vi "Test_uart.vi"() -> ()   [LabVIEW 2025]
uses:
  <vilib>/Instr/_visa.llb/VISA Configure Serial Port (Instr).vi
panel:
  in  "Caja engranes":sgl
  in  "Stop Button":bool
  out "Waveform Chart":cluster{"Número":sgl, "Número":sgl}(graph)
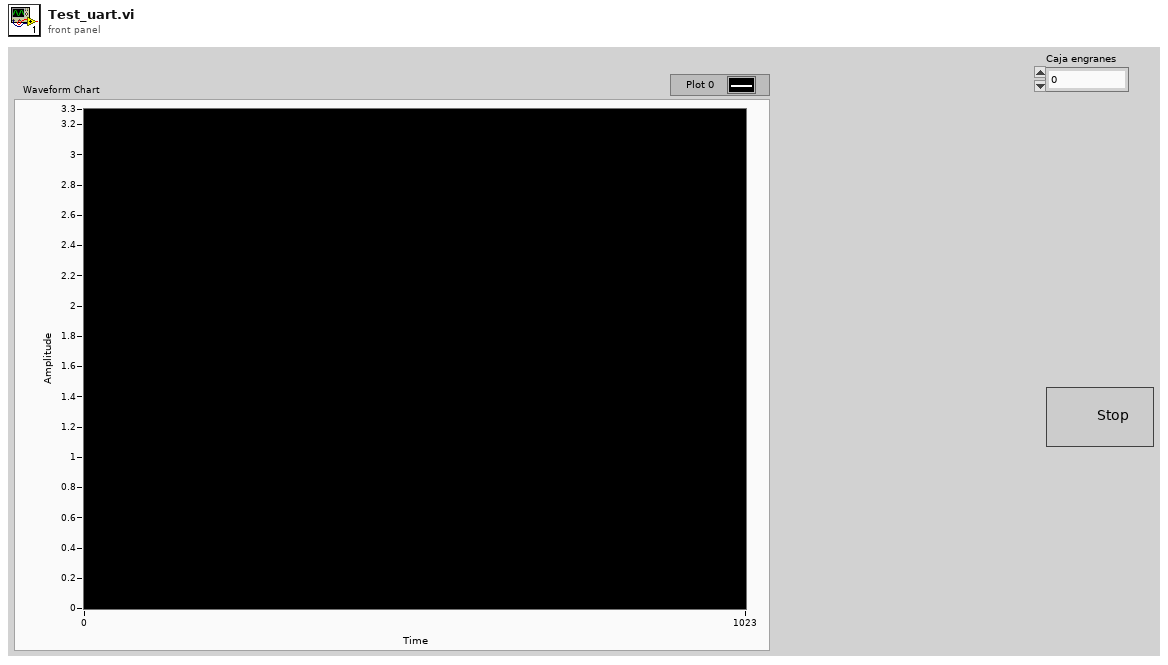
[diagram p1: front panel]
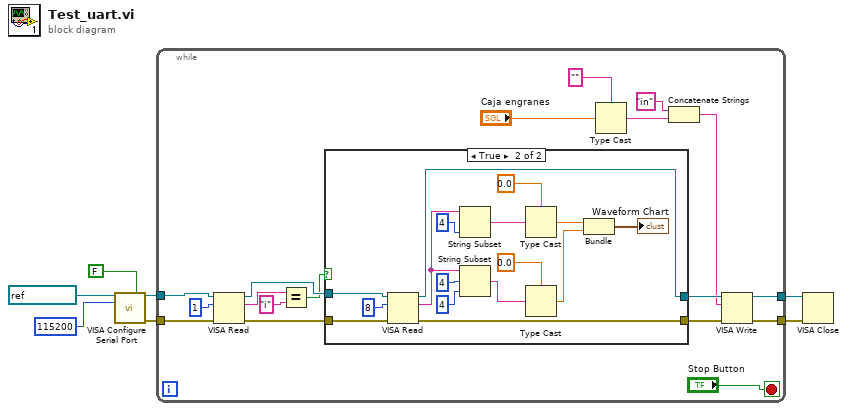
[diagram p0: block diagram]
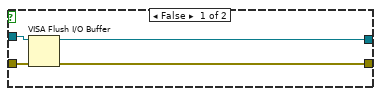
[diagram p2: hidden frame]
diagram:
  n1 = call-poly "VISA Configure Serial Port"("VISA resource name"=refnum<visa-resource-name> "COM14", "Enable Termination\nChar (T)"=FALSE ("Enable Termination\nChar (T)"), "baud rate (9600)"=u32 115200) -> ("VISA resource name out"=w2:refnum<visa-resource-name>, "error out"=w1:errorcluster)  [unwired: 11 in]
  n2 = while {
    tunnel: w2 -> [w23]
    tunnel: w1 -> [w22]
    tunnel: [w13] -> w7
    tunnel: [w14] -> w6
    stop <- "Stop Button" stop-if-true
    n3 = VISA Read(VISA resource name=w23, byte count=u32 1, error in (no error)=w22) -> (VISA resource name out=w21:refnum<visa-resource-name>, read buffer=w19:string, error out=w20:errorcluster)  [unwired: 1 out]
    n4 = Equal?(x=w19, y="i") -> (x = y?=w17:bool)
    n5 = case shown="True" w17 {
      tunnel: [w29 w45] -> w12
      tunnel: [w28 w44] -> w11
      tunnel: w21 -> [w27 w41]
      tunnel: w20 -> [w26 w40]
      frame False {
        n6 = VISA Flush I/O Buffer(VISA resource name=w27, error in (no error)=w26) -> (VISA resource name out=w29:refnum<visa-resource-name>, error out=w28:errorcluster)  [unwired: 1 in]
      }
      frame True {
        n7 = VISA Read(VISA resource name=w41, byte count=u32 8, error in (no error)=w40) -> (VISA resource name out=w45:refnum<visa-resource-name>, read buffer=w36:string, error out=w44:errorcluster)  [unwired: 1 out]
        n8 = String Subset(string=w36, length (rest)=4 ("length (rest)")) -> (substring=w38:string)  [unwired: 1 in]
        n9 = String Subset(string=w36, offset (0)=4, length (rest)=4 ("length (rest)")) -> (substring=w30:string)
        n10 = Type Cast(type=sgl 0.0 ("Número"), x=w38) -> (*(type *) &x=w34:sgl)
        n11 = Type Cast(type=sgl 0.0 ("Número"), x=w30) -> (*(type *) &x=w31:sgl)
        n12 = Bundle("Número"=w34, "Número"=w31) -> (→"Waveform Chart":cluster{"Número":sgl, "Número":sgl})  [unwired: 1 in]
      }
    }
    n13 = Type Cast(type="", x="Caja engranes") -> (*(type *) &x=w9:string)
    n14 = Concatenate Strings("in", w9) -> (w8:string)
    n15 = VISA Write(VISA resource name=w12, write buffer=w8, error in (no error)=w11) -> (VISA resource name out=w13:refnum<visa-resource-name>, error out=w14:errorcluster)  [unwired: 1 out]
  }
  n16 = VISA Close(VISA resource name=w7, error in (no error)=w6) -> ()  [unwired: 1 out]
